vi "thickness_recognize.vi"(8 "干涉宽度":u32, 9 "干涉阈值":dbl, 10 "A":dbl[](array[numeric]), 11 "S":dbl[](array[numeric])) -> (0 "添加的数组":i32[](array[numeric]), 2 "MAX_Index":i32, 3 "INDEX":i32[](array[numeric]))   [LabVIEW 2015, in "Boimetry Processing.lvlib"]
uses:
  Boimetry Processing.lvlib
  <vilib>/Analysis/NI_AALPro.lvlib
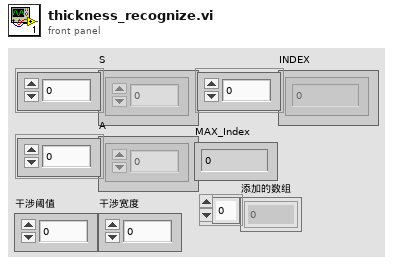
[diagram p1: front panel]
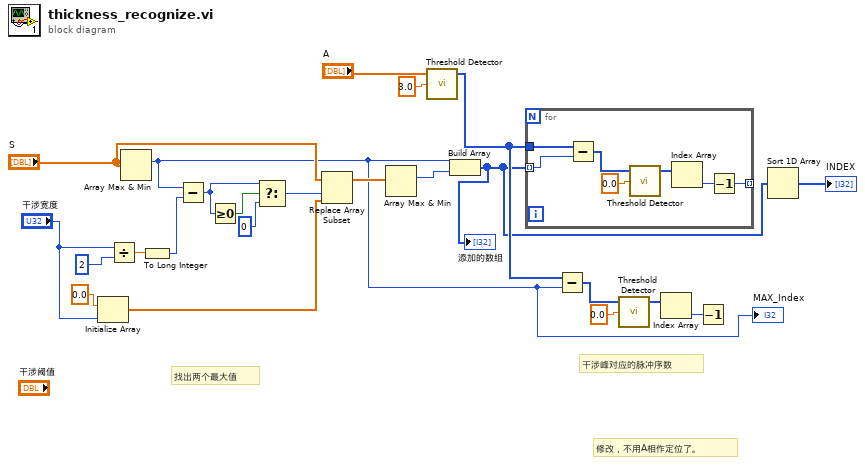
[diagram p0: block diagram]
diagram:
  # "修改，不用A相作定位了。"
  # "找出两个最大值"
  # "干涉峰对应的脉冲序数"
  n1 = Initialize Array(0.0 ("元素"), "干涉宽度") -> (w18:dbl[])
  n2 = Divide(x="干涉宽度", y=u32 2) -> (x/y=w22:dbl)
  n3 = Array Max & Min(array="S") -> (max index (indices)=w1:i32)  [unwired: 3 out]
  "MAX_Index" <- w1
  n4 = To Long Integer(number=w22) -> (32bit integer=w21:i32)
  n5 = Subtract(x=w1, y=w21) -> (x-y=w8:i32)
  n6 = Greater Or Equal To 0?(x=w8) -> (x >= 0?=w9:bool)
  n7 = Select(t=w8, s=w9, f=u32 0) -> (s? t:f=w6:u32)
  n8 = Replace Array Subset(array="S", new element=w18, index=w6) -> (w5:dbl[])
  n9 = Array Max & Min(array=w5) -> (max index (indices)=w17:i32)  [unwired: 3 out]
  n10 = call <vilib>:"Threshold Detector.vi"("threshold"=3.0, "X"="A") -> ("Indices"=w10:i32[])  [unwired: 1 in, 2 out]
  n11 = Build Array(w1, w17) -> (w2:i32[])
  "添加的数组" <- w2
  n12 = for {
    tunnel: w2 -> [w30] mode=indexing
    tunnel: w10 -> [w26]
    tunnel: [w24] -> _ mode=indexing
    n13 = Subtract(x=w26, y=w30) -> (x-y=w28:i32[])
    n14 = call <vilib>:"Threshold Detector.vi"("threshold"=0.0, "X"=w28) -> ("Indices"=w27:i32[])  [unwired: 1 in, 2 out]
    n15 = Index Array(array=w27) -> (element=w25:i32)  [unwired: 1 in]
    n16 = Decrement(x=w25) -> (x-1=w24:i32)
  }
  n17 = Subtract(x=w10, y=w1) -> (x-y=w13:i32[])
  n18 = call <vilib>:"Threshold Detector.vi"("threshold"=0.0, "X"=w13) -> ("Indices"=w12:i32[])  [unwired: 1 in, 2 out]
  n19 = Index Array(array=w12) -> (element=w11:i32)  [unwired: 1 in]
  n20 = Decrement(x=w11) -> ()  [unwired: 1 out]
  n21 = Sort 1D Array(array=w2) -> (sorted array=→"INDEX":i32[])
